vi "main.vi"() -> ()   [LabVIEW 2013]
uses:
  <vilib>/Utility/error.llb/whitespace.ctl
panel:
  in  "质量产品ID":string="201308280001" caption="产品ID"
  out "设备号字符":string
  in  "合格":bool
  in  "设备号":u16(ring)=1 items=["00", "01", "02", "03", "04", "05", "06", "07", "08", "09", "10", "11", "12", "13", "14"]
  in  "写入合格":bool
  # "手动写入质量数据"
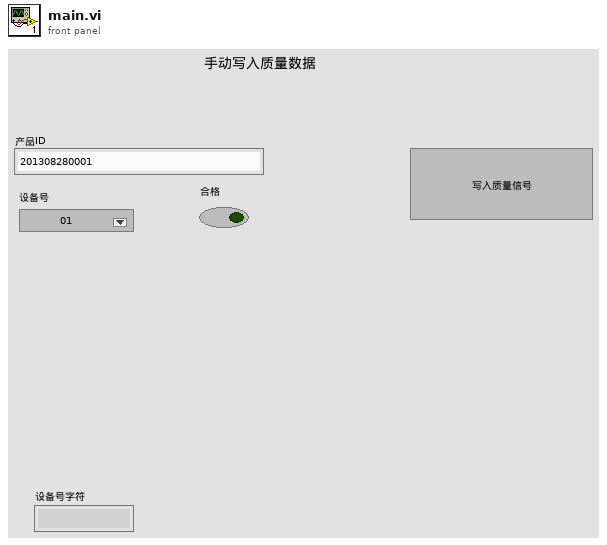
[diagram p1: front panel]
types:
  T1 = typedef "whitespace.ctl" = u16
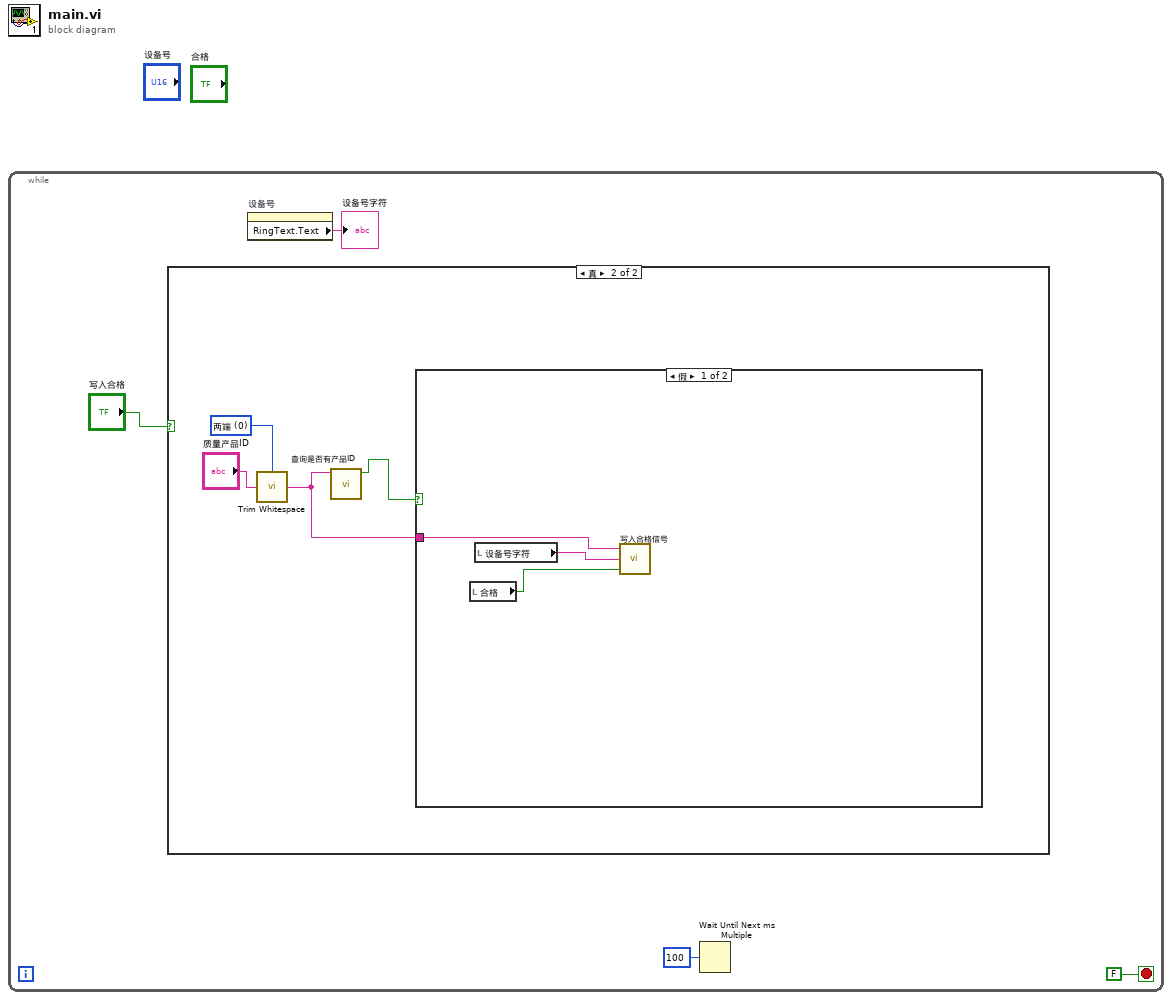
[diagram p0: block diagram]
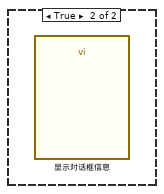
[diagram p3: hidden frame]
diagram:
  n1 = while {
    stop <- FALSE stop-if-true
    n2 = case shown="真" "写入合格" {
      frame False {
      }
      frame True {
        w8 = T1 0 items=["两端", "字符串首端", "字符串末端"] ("location (both)")
        n3 = call <vilib>:"Trim Whitespace.vi"("string"="质量产品ID", "location (both)"=w8) -> ("trimmed string"=w5:string)
        n4 = call "查询是否有产品ID.vi"("转向器总成ID"=w5) -> ("无重号"=w6:bool)  [unwired: 9 in, 1 out]
        n5 = case shown="假" w6 {
          tunnel: w5 -> [w11 _]
          frame False {
            n6 = local read "合格"() -> (w9:bool)
            n7 = local read "设备号字符"() -> (w10:string)
            n8 = call "写入合格信号.vi"("信号"=w9, "设备号"=w10, "产品ID"=w11) -> ()  [unwired: 2 in]
          }
          frame True {
            n9 = call "显示对话框信息"() -> ()  [unwired: 10 in, 2 out]
          }
        }
      }
    }
    n10 = property on="设备号" class="Ring (严格)"() -> ("RingText.Text"=→"设备号字符":string)  [unwired: 2 in, 2 out]
    n11 = Wait Until Next ms Multiple(millisecond multiple=u32 100 ("毫秒倍数")) -> ()  [unwired: 1 out]
  }
